vi "Update DUT Pass Fail.vi"(8 "error in (no error)":errorcluster, 9 "Position":u32, 10 "Test Passed":bool, 11 "Application in":refnum<class "Application.lvclass">) -> (0 "error out":errorcluster, 3 "Application out":refnum<class "Application.lvclass">)   [LabVIEW 2017, in "Application.lvlib" / "Application.lvclass"]
doc: "If a position is running and already passed, this vi will update the position with the new status. If it has already failed, it ignores the test passed boolean and keeps the position failed. If the board is not Running or Failed this vi ignores the inputs."
uses:
  Application.lvclass
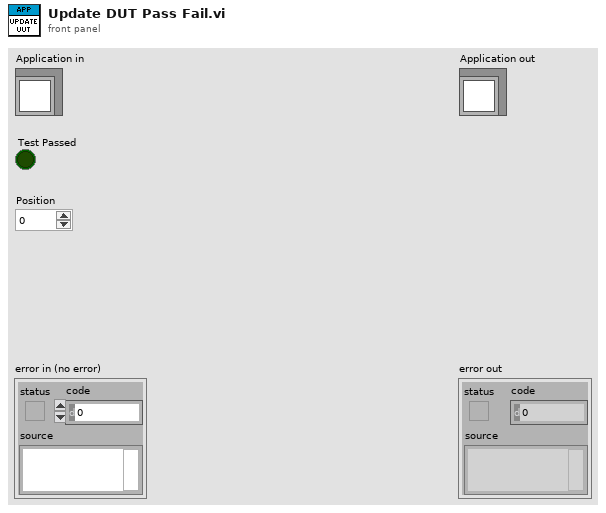
[diagram p1: front panel]
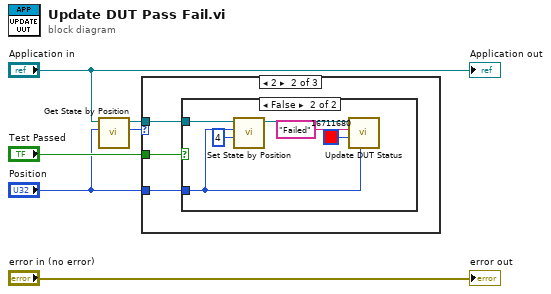
[diagram p0: block diagram]
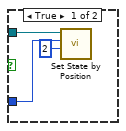
[diagram p3: hidden frame]
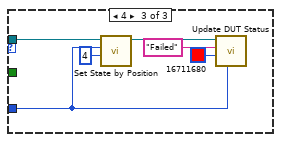
[diagram p4: hidden frame]
diagram:
  n1 = call-dynamic "Get State by Position.vi"("Position"="Position", "Application in"="Application in") -> ("State"=w5:u32, "Application out"=w1:refnum<class "Application.lvclass">)  [unwired: 7 in, 1 out]
  n2 = case shown="2" w5 {
    tunnel: "Test Passed" -> [_ w9 _]
    tunnel: "Position" -> [_ w8 w19]
    tunnel: w1 -> [_ w7 w20]
    frame Default {
    }
    frame 2 {
      n3 = case shown="False" w9 {
        tunnel: w8 -> [w10 w14]
        tunnel: w7 -> [w11 w13]
        frame True {
          n4 = call-dynamic "Set State by Position.vi"("State"=u32 2, "Position"=w10, "Application in"=w11) -> ()  [unwired: 7 in, 2 out]
        }
        frame False {
          n5 = call-dynamic "Set State by Position.vi"("State"=u32 4, "Position"=w14, "Application in"=w13) -> ("Application out"=w17:refnum<class "Application.lvclass">)  [unwired: 7 in, 1 out]
          n6 = call "Update DUT Status.vi"("Position"=w14, "BG Color"=u32 16711680, "Message ('')"="Failed", "Application in"=w17) -> ()  [unwired: 6 in, 2 out]
        }
      }
    }
    frame 4 {
      n7 = call-dynamic "Set State by Position.vi"("State"=u32 4, "Position"=w19, "Application in"=w20) -> ("Application out"=w23:refnum<class "Application.lvclass">)  [unwired: 7 in, 1 out]
      n8 = call "Update DUT Status.vi"("Position"=w19, "BG Color"=u32 16711680, "Message ('')"="Failed", "Application in"=w23) -> ()  [unwired: 6 in, 2 out]
    }
  }
  "error out" <- "error in (no error)"
  "Application out" <- "Application in"
